vi "Autonomous Independent.vi"() -> ()   [LabVIEW 2017]
doc: "This VI is called when autonomous begins, and will automatically be terminated when autonomous ends. You can carry out timed or sensor driven robot movement independently without needing to return to the caller."
uses:
  <vilib>/Rock Robotics/WPI/ThirdParty/Phoenix-LabVIEW/Motor Controller/Controls/CTRE_Phoenix_MotorControl_FeedbackDevice.ctl
  <vilib>/Rock Robotics/WPI/ThirdParty/Phoenix-LabVIEW/Motor Controller/Controls/CTRE_Phoenix_MotorControl_StatusFrameEnhanced.ctl
  <vilib>/Rock Robotics/WPI/ThirdParty/Phoenix-LabVIEW/Motor Controller/Controls/CTRE_Phoenix_MotorControl_ControlMode.ctl
  <vilib>/Rock Robotics/WPI/ThirdParty/Phoenix-LabVIEW/Motor Controller/Controls/CTRE_Phoenix_MotorControl_TrajectoryPointTimeDur.ctl
  <vilib>/Utility/file.llb/Read Delimited Spreadsheet (DBL).vi
panel:
  out "Velocity (Sensor Units per 100 ms)":i32
  out "Position (Sensor Units)":i32
  out "Loop Time":u32
  out "Is Last?":bool
  out "Active Point Valid?":bool
  out "Is Underrun?":bool
  out "Has Underrun?":bool
  out "Top Buffer Count":i32
  out "Bottom Buffer Count":i32
  # "Be sure to right-click and choose Data Operations>>Make Current Value default if you want to save the array values with the VI"
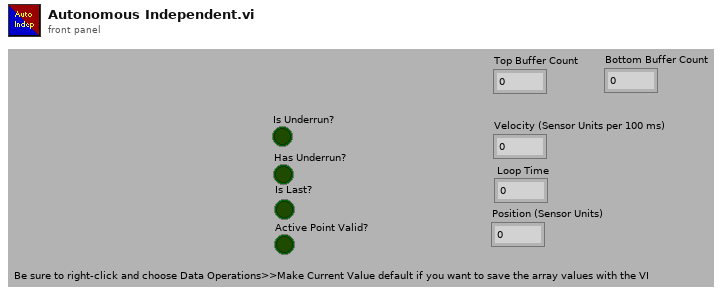
[diagram p1: front panel]
types:
  T1 = typedef "CTRE_Phoenix_MotorControl_StatusFrameEnhanced.ctl" = u16
  T2 = typedef "CTRE_Phoenix_MotorControl_FeedbackDevice.ctl" = i8
  T3 = typedef "WPI_MotorControlDeviceRef.ctl" = cluster{"DeviceStatus":errorcluster, "Type":T4, "PWM":cluster{"PWM Channel":T5, "DeadBand":T6}, "CAN":cluster{"Device Number":u8, "SetOutput VI Ref":variant, "GetOutput VI Ref":variant, "Enable VI Ref":variant, "Disable VI Ref":variant, "Data":variant}, "Invert":bool, "DIO PWM":cluster{"PWM \"Enable\" Channel":T5, "DIOChannel":T7, "PWM Rate":dbl}}
  T4 = typedef "WPI_MotorControlType.ctl" = enum16{"PWM", "CAN", "DIO PWM"}
  T5 = typedef "FPGA_DIOPWMChannel.ctl" = enum8{"PWM 0", "PWM 1", "PWM 2", "PWM 3", "PWM 4", "PWM 5", "PWM 6", "PWM 7", "PWM 8", "PWM 9", "PWM MXP 0", "PWM MXP 1", "PWM MXP 2", "PWM MXP 3", "PWM MXP 4", "PWM MXP 5", "PWM MXP 6", "PWM MXP 7", "PWM MXP 8", "PWM MXP 9", "Invalid"}
  T6 = typedef "WPI_PWMDeadband.ctl" = cluster{"Name":string, "maxPositivePwm":i32, "minPositivePwm":i32, "centerPwm":i32, "maxNegativePwm":i32, "minNegativePwm":i32, "angularRange":u16}
  T7 = typedef "FPGA_DIOChannel.ctl" = enum8{"DIO 0", "DIO 1", "DIO 2", "DIO 3", "DIO 4", "DIO 5", "DIO 6", "DIO 7", "DIO 8", "DIO 9", "DIO MXP 0", "DIO MXP 1", "DIO MXP 2", "DIO MXP 3", "DIO MXP 4", "DIO MXP 5", "DIO MXP 6", "DIO MXP 7", "DIO MXP 8", "DIO MXP 9", "DIO MXP 10", "DIO MXP 11", "DIO MXP 12", "DIO MXP 13", "DIO MXP 14", "DIO MXP 15", "SPI Port CS1", "SPI Port CS2", "SPI Port CS3", "SPI Port MISO", "SPI Port MOSI", "Invalid"}
  T8 = typedef "CTRE_Phoenix_MotorControl_ControlMode.ctl" = u16
  T9 = cluster{"Top Buffer Remaining":i32, "Top Buffer Count":i32, "Bottom Buffer Count":i32, "Has Underrun?":bool, "Is Underrun?":bool, "Active Point Valid?":bool, "Is Last?":bool, "Profile Slot Select 0":i32, "Output Enable":i32, "Time Duration (ms)":i32, "Profile Slot Select 1":i32}
  T10 = typedef "CTRE_Phoenix_MotorControl_TrajectoryPointTimeDur.ctl" = i32
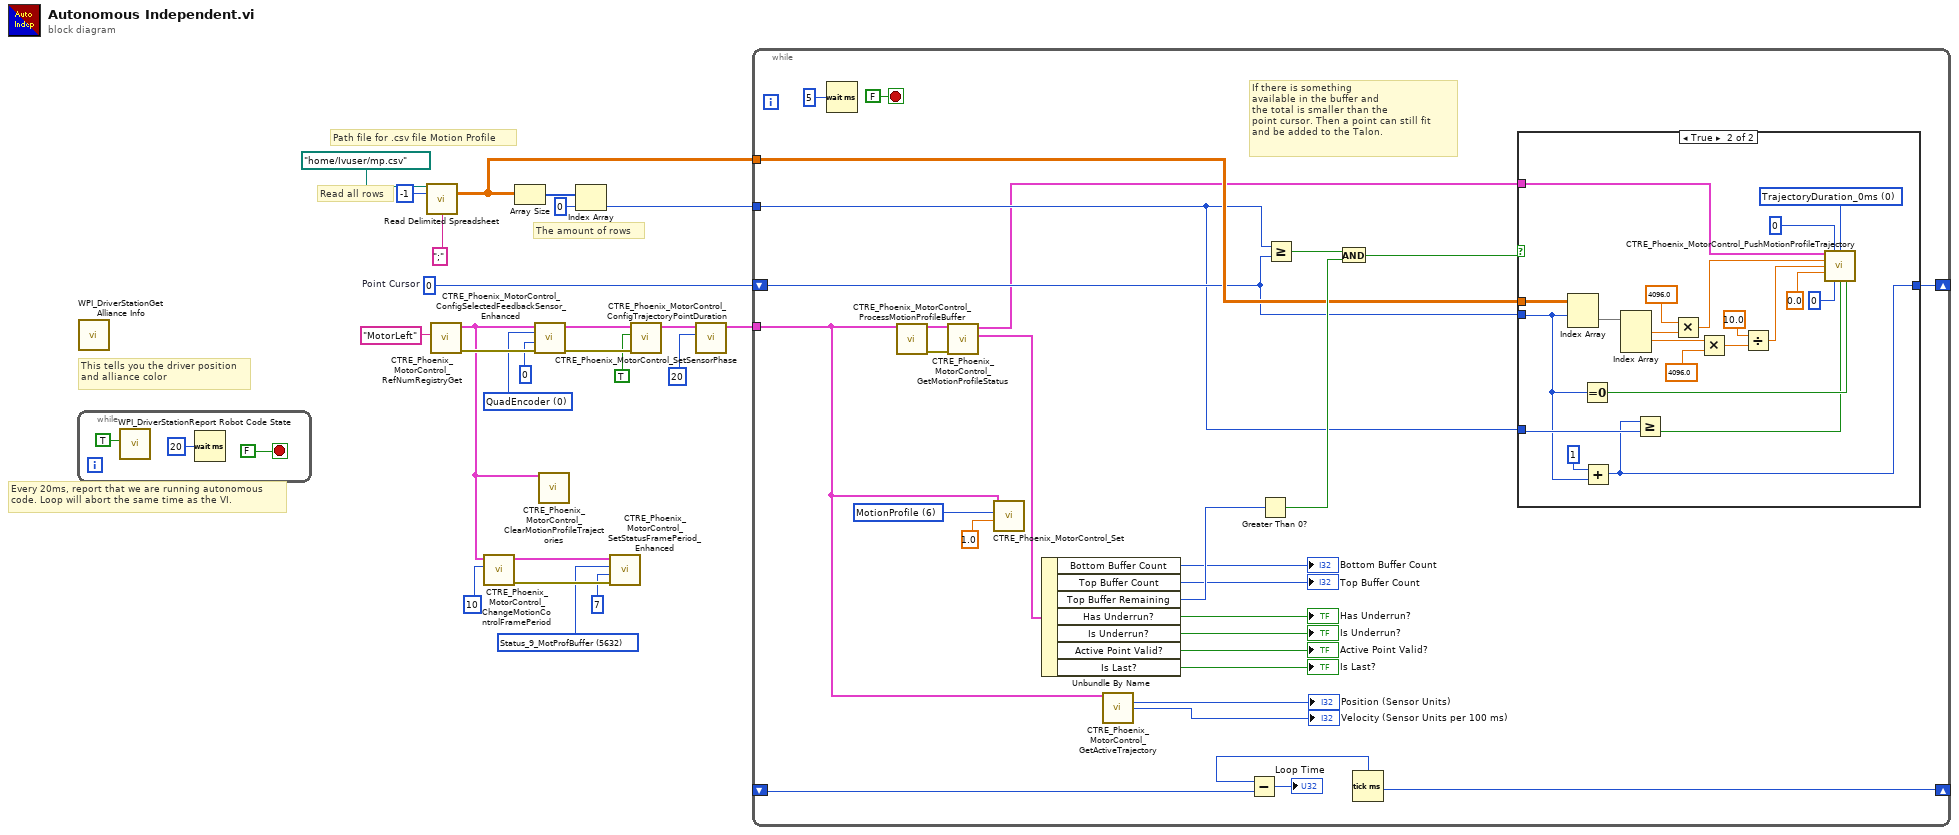
[diagram p0: block diagram]
diagram:
  w2 = 0  # Point Cursor
  w11 = T1 5632 items=["Status_1_General"=5120, "Status_2_Feedback0"=5184, "Status_3_Quadrature"=5248, "Status_4_AinTempVbat"=5312, "Status_6_Misc"=5440, "Status_7_CommStatus"=5504, "Status_8_PulseWidth"=5568, "Status_9_MotProfBuffer"=5632, "Status_10_MotionMagic"=5696, "Status_11_UartGadgeteer"=5760, "Status_12_Feedback1"=5824, "Status_13_Base_PIDF0"=5888, "Status_14_Turn_PIDF1"=5952, "Status_15_FirmwareApiStatus"=6016] ("Status Frame")
  w21 = T2 0 items=["None"=-1, "QuadEncoder"=0, "Analog"=2, "Tachometer"=4, "Pulse Width Encoded Position"=8, "Sensor Sum (S0 + S1)"=9, "Sensor Difference (D0 - D1)"=10, "Remote Source 0"=11, "Remote Source 1"=12, "Software Emulated"=15] ("Feedback Device")
  # "The amount of rows"
  # "Path file for .csv file Motion Profile"
  # "Read all rows"
  # "Every 20ms, report that we are running autonomous\ncode. Loop will abort the same time as the VI."
  # "This tells you the driver position\nand alliance color"
  n1 = while {
    stop <- FALSE stop-if-true
    n2 = call <vilib>:"WPI_DriverStationReport Robot Code State.vi"("Autonomous"=TRUE) -> ()  [unwired: 10 in, 1 out]
    n3 = Wait (ms)(milliseconds to wait=u32 20) -> ()  [unwired: 1 out]
  }
  n4 = call <vilib>:"WPI_DriverStationGet Alliance Info.vi"() -> ()  [unwired: 12 out]
  n5 = call-poly <vilib>:"Read Delimited Spreadsheet.vi"("file path (dialog if empty)"=path "/home/Ivuser/mp.csv", "number of rows (all:-1)"=-1, "delimiter (\\t)"=";" ("delimiter (\\t)")) -> ("all rows"=w4:dbl[][])  [unwired: 7 in, 5 out]
  n6 = call <vilib>:"CTRE_Phoenix_MotorControl_RefNumRegistryGet.vi"("refnum name"="MotorLeft") -> ("error out"=w23:errorcluster, "PhoenixMotorControlDevRef"=w1:T3)  [unwired: 9 in]
  n7 = call <vilib>:"CTRE_Phoenix_MotorControl_ChangeMotionControlFramePeriod.vi"("periodMs"=10, "PhoenixMotorControlDevRef"=w1) -> ("error out"=w12:errorcluster, "PhoenixMotorControlDevRef"=w13:T3)  [unwired: 8 in]
  n8 = Array Size(array=w4) -> (size(s)=w8:i32[])
  n9 = call <vilib>:"CTRE_Phoenix_MotorControl_ConfigSelectedFeedbackSensor_Enhanced.vi"("error in (no error)"=w23, "pidLoopIdx"=0, "Feedback Device"=w21, "PhoenixMotorControlDevRef"=w1) -> ("error out"=w19:errorcluster, "PhoenixMotorControlDevRef"=w20:T3)  [unwired: 6 in]
  n10 = call <vilib>:"CTRE_Phoenix_MotorControl_ClearMotionProfileTrajectories.vi"("PhoenixMotorControlDevRef"=w1) -> ()  [unwired: 13 in, 2 out]
  n11 = Index Array(array=w8, index=0) -> (element=w3:i32)
  n12 = call <vilib>:"CTRE_Phoenix_MotorControl_SetStatusFramePeriod_Enhanced.vi"("error in (no error)"=w12, "periodMs"=7, "Status Frame"=w11, "PhoenixMotorControlDevRef"=w13) -> ()  [unwired: 6 in, 2 out]
  n13 = call <vilib>:"CTRE_Phoenix_MotorControl_SetSensorPhase.vi"("error in (no error)"=w19, "PhaseSensor"=TRUE, "PhoenixMotorControlDevRef"=w20) -> ("PhoenixMotorControlDevRef"=w17:T3)  [unwired: 7 in, 1 out]
  n14 = call <vilib>:"CTRE_Phoenix_MotorControl_ConfigTrajectoryPointDuration.vi"("durationMs"=20, "PhoenixMotorControlDevRef"=w17) -> ("PhoenixMotorControlDevRef"=w15:T3)  [unwired: 8 in, 1 out]
  n15 = while {
    tunnel: w4 -> [w47]
    tunnel: w3 -> [w45]
    tunnel: w15 -> [w28]
    shift-right: [w43] -> _
    shift-left: w2 -> [w46]
    shift-right: [w35] -> _
    shift-left: _ -> [w36]
    stop <- FALSE stop-if-true
    w30 = T8 6 items=["PercentOutput"=0, "Position"=1, "Velocity"=2, "Current"=3, "Follower"=5, "MotionProfile"=6, "MotionMagic"=7, "MotionMagicArc"=8, "MotionProfileArc"=10, "Disabled"=15] ("Control Mode")
    # "If there is something\navailable in the buffer and\nthe total is smaller than the\npoint cursor. Then a point can still fit\nand be added to the Talon."
    n16 = Wait (ms)(milliseconds to wait=u32 5) -> ()  [unwired: 1 out]
    n17 = call <vilib>:"CTRE_Phoenix_MotorControl_ProcessMotionProfileBuffer.vi"("PhoenixMotorControlDevRef"=w28) -> ("PhoenixMotorControlDevRef"=w52:T3, "error out"=w53:errorcluster)  [unwired: 13 in]
    n18 = call <vilib>:"CTRE_Phoenix_MotorControl_GetMotionProfileStatus.vi"("error in"=w53, "PhoenixMotorControlDevRef"=w52) -> ("Motion Profile Status"=w51:T9, "PhoenixMotorControlDevRef"=w31:T3)  [unwired: 7 in, 1 out]
    n19 = call <vilib>:"CTRE_Phoenix_MotorControl_Set.vi"("Output"=1.0, "Control Mode"=w30, "PhoenixMotorControlDevRef"=w28) -> ()  [unwired: 7 in, 2 out]
    n20 = Unbundle By Name(w51) -> ("Bottom Buffer Count"=→"Bottom Buffer Count":i32, "Top Buffer Count"=→"Top Buffer Count":i32, "Top Buffer Remaining"=w44:i32, "Has Underrun?"=→"Has Underrun?":bool, "Is Underrun?"=→"Is Underrun?":bool, "Active Point Valid?"=→"Active Point Valid?":bool, "Is Last?"=→"Is Last?":bool)
    n21 = call <vilib>:"CTRE_Phoenix_MotorControl_GetActiveTrajectory.vi"("PhoenixMotorControlDevRef"=w28) -> ("Position (Sensor Units)"=→"Position (Sensor Units)":i32, "Velocity (Sensor Units per 100 ms)"=→"Velocity (Sensor Units per 100 ms)":i32)  [unwired: 10 in, 3 out]
    n22 = Greater Than 0?(x=w44) -> (x > 0?=w49:bool)
    n23 = Greater Or Equal?(x=w45, y=w46) -> (x >= y?=w50:bool)
    n24 = And(x=w50, y=w49) -> (x .and. y?=w48:bool)
    n25 = Tick Count (ms)() -> (millisecond timer value=w35:u32)
    n26 = Subtract(x=w35, y=w36) -> (x-y=→"Loop Time":u32)
    n27 = case shown="True" w48 {
      tunnel: w47 -> [_ w77]
      tunnel: w46 -> [w56 w64]
      tunnel: w45 -> [_ w65]
      tunnel: w31 -> [_ w62]
      tunnel: [w56 w61] -> w43
      frame False {
      }
      frame True {
        w57 = T10 0 items=["TrajectoryDuration_0ms"=0, "TrajectoryDuration_5ms"=5, "TrajectoryDuration_10ms"=10, "TrajectoryDuration_20ms"=20, "TrajectoryDuration_30ms"=30, "TrajectoryDuration_40ms"=40, "TrajectoryDuration_50ms"=50, "TrajectoryDuration_100ms"=100] ("durationMs")
        n28 = Index Array(array=w77, index (row)=w64) -> (element=w76:dbl[])  [unwired: 1 in]
        n29 = Equal To 0?(x=w64) -> (x = 0?=w67:bool)
        n30 = Add(x=1, y=w64) -> (x+y=w61:i32)
        n31 = Index Array(array=w76) -> (element #1=w75:dbl, element #2=w73:dbl)  [unwired: 3 in, 1 out]
        n32 = Greater Or Equal?(x=w61, y=w65) -> (x >= y?=w63:bool)
        n33 = Multiply(x=4096.0 ("element"), y=w75) -> (x*y=w69:dbl)
        n34 = Multiply(x=w73, y=4096.0) -> (x*y=w71:dbl)
        n35 = Divide(x=10.0, y=w71) -> (x/y=w68:dbl)
        n36 = call <vilib>:"CTRE_Phoenix_MotorControl_PushMotionProfileTrajectory.vi"("PhoenixMotorControlDevRef"=w62, "profileSlotSelect1"=0, "durationMs"=w57, "position"=w69, "velocity"=w68, "auxiliaryPos"=0.0, "profileSlotSelect0"=0, "isLastPoint?"=w63, "Zero Position?"=w67) -> ()  [unwired: 5 in, 2 out]
      }
    }
  }
